vi "Cleanup Resource DB.vi"(8 "error in (no error)":errorcluster, 11 "ProjectData in":refnum<class "Project Data.lvclass">) -> (0 "error out":errorcluster, 3 "ProjectData out":refnum<class "Project Data.lvclass">)   [LabVIEW 2013, in "SET Project Data.lvlib" / "Project Data.lvclass"]
uses:
  Project Data.lvclass
  Project Data.lvclass/Project Data.ctl
  Types/ProjFile_Resource Entry.ctl
  Resource Data Class/Resource Data.lvclass/Resource Data.ctl
  Resource Data Class/Resource Data.lvclass
  Resource Data Class/Read Resources.vi
  VI Class/VI Data.lvclass
  Menu Class/Menu Data.lvclass
  SET Project Data.lvlib
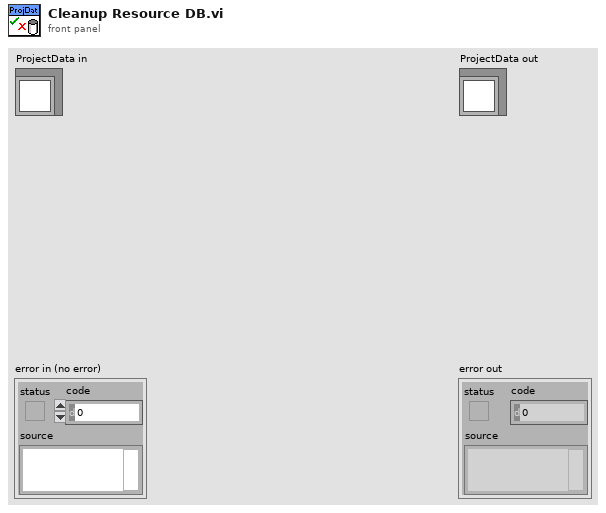
[diagram p1: front panel]
types:
  T1 = typedef "SET Project Data.lvlib/ProjFile_Resource Entry.ctl" = cluster{"RID":string, "Tag":string, "Strings [] (UTF-16)":string[], "Shared?":bool}
  T2 = typedef "SET Project Data.lvlib/ProjFile_VI Data.ctl" = cluster{"VI Path":path, "GObjects[]":T3[]}
  T3 = typedef "SET Project Data.lvlib/ProjFile_GObject Data.ctl" = cluster{"UID":i32, "Label":string, "ClassName":string, "Item List[]":cluster{"Item Name":string, "RID":string}[]}
  T4 = typedef "SET Project Data.lvlib/ProjFile_Menu Data.ctl" = cluster{"Menu Path":path, "Menu Items[]":cluster{"Tag":string, "RID":string}[]}
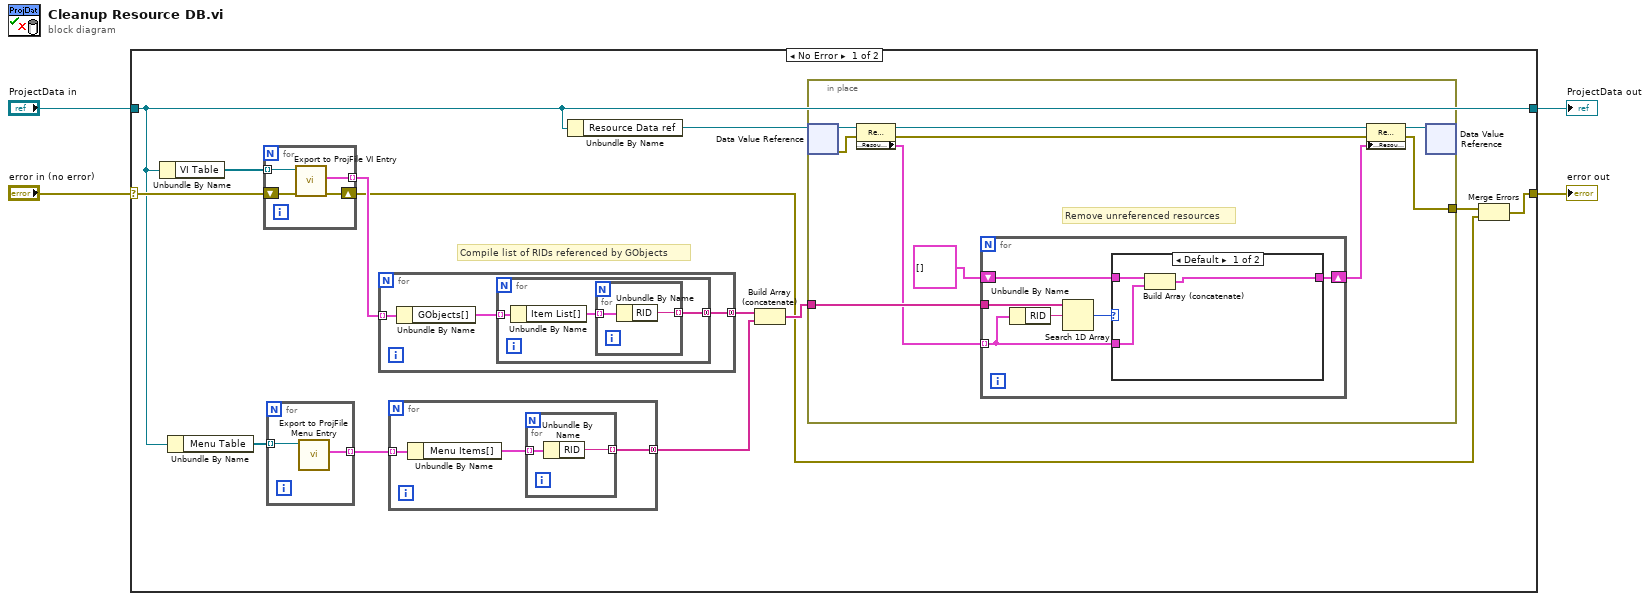
[diagram p0: block diagram]
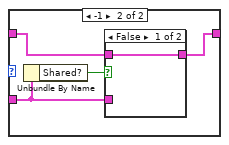
[diagram p2: hidden frame]
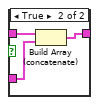
[diagram p3: hidden frame]
diagram:
  n1 = case shown="No Error" "error in (no error)" {
    selector: "error in (no error)" -> [w15 w65]
    tunnel: [w6 w65] -> w3
    tunnel: [w14 w64] -> w1
    tunnel: "ProjectData in" -> [w14 w64]
    frame No Error {
      # "Compile list of RIDs referenced by GObjects"
      n2 = Unbundle By Name(w14) -> ("VI Table"=w17:refnum<class "VI Data.lvclass">[])
      n3 = Unbundle By Name(w14) -> ("Menu Table"=w13:refnum<class "Menu Data.lvclass">[])
      n4 = for {
        shift-right: [w63] -> w5
        shift-left: w15 -> [w62]
        tunnel: w17 -> [w61] mode=indexing
        tunnel: [w60] -> w16 mode=indexing
        n5 = call "Export to ProjFile VI Entry.vi"("error in (no error)"=w62, "LanguageData in"=w61) -> ("error out"=w63:errorcluster, "VI Data"=w60:T2)  [unwired: 7 in, 1 out]
      }
      n6 = for {
        tunnel: w13 -> [w51] mode=indexing
        tunnel: [w50] -> w12 mode=indexing
        n7 = call "Export to ProjFile Menu Entry.vi"("Menu Data in"=w51) -> ("Menu Data"=w50:T4)  [unwired: 8 in, 2 out]
      }
      n8 = for {
        tunnel: w16 -> [w54] mode=indexing
        tunnel: [w52] -> w11 mode=concatenating
        n9 = Unbundle By Name(w54) -> ("GObjects[]"=w53:T3[])
        n10 = for {
          tunnel: w53 -> [w57] mode=indexing
          tunnel: [w55] -> w52 mode=concatenating
          n11 = Unbundle By Name(w57) -> ("Item List[]"=w56:cluster{"Item Name":string, "RID":string}[])
          n12 = for {
            tunnel: w56 -> [w59] mode=indexing
            tunnel: [w58] -> w55 mode=indexing
            n13 = Unbundle By Name(w59) -> ("RID"=w58:string)
          }
        }
      }
      n14 = for {
        tunnel: w12 -> [w47] mode=indexing
        tunnel: [w45] -> w10 mode=concatenating
        n15 = Unbundle By Name(w47) -> ("Menu Items[]"=w46:cluster{"Tag":string, "RID":string}[])
        n16 = for {
          tunnel: w46 -> [w49] mode=indexing
          tunnel: [w48] -> w45 mode=indexing
          n17 = Unbundle By Name(w49) -> ("RID"=w48:string)
        }
      }
      n18 = Unbundle By Name(w14) -> ("Resource Data ref"=w8:refnum<data-value>)
      n19 = Build Array (concatenate)(w11, w10) -> (w9:string[])
      n20 = in-place {
        in-place-border: w9 -> [w27]
        in-place-border: [w23] -> w7
        # "Remove unreferenced resources"
        n21 = in-place-dvr #1(w8) -> (w25:refnum<class "Resource Data.lvclass">, w18:errorcluster)
        n22 = property class="Resource Data.lvclass"(reference=w25, error in=w18) -> (reference out=w20:refnum<class "Resource Data.lvclass">, error out=w19:errorcluster, "Properties:Resources []"=w24:T1[])
        n23 = for {
          tunnel: w27 -> [w33]
          tunnel: w24 -> [w30] mode=indexing
          shift-right: [w28] -> w21
          shift-left: T1[] [] ("Resources []") -> [w29]
          n24 = Unbundle By Name(w30) -> ("RID"=w32:string)
          n25 = Search 1D Array(1D array=w33, element=w32) -> (index of element=w31:i32)  [unwired: 1 in]
          n26 = case shown="Default" w31 {
            tunnel: w30 -> [w36 w39]
            tunnel: w29 -> [w35 w38]
            tunnel: [w34 w37] -> w28
            frame Default {
              n27 = Build Array (concatenate)(w35, w36) -> (w34:T1[])
            }
            frame -1 {
              n28 = Unbundle By Name(w39) -> ("Shared?"=w40:bool)
              n29 = case shown="False" w40 {
                tunnel: w39 -> [_ w43]
                tunnel: w38 -> [w41 w44]
                tunnel: [w41 w42] -> w37
                frame False {
                }
                frame True {
                  n30 = Build Array (concatenate)(w44, w43) -> (w42:T1[])
                }
              }
            }
          }
        }
        n31 = property class="Resource Data.lvclass"(reference=w20, error in=w19, "Properties:Resources []"=w21) -> (reference out=w22:refnum<class "Resource Data.lvclass">, error out=w23:errorcluster)
        n32 = in-place-dvr #1(w22) -> ()  [unwired: 2 out]
      }
      n33 = Merge Errors(w7, w5) -> (w6:errorcluster)
    }
    frame Error {
    }
  }
  "error out" <- w3
  "ProjectData out" <- w1
